vi "Refresh All Hightlight.vi"(0 "Display State In":T1={"logTable"=refnum, "max items"=500, "displaydata"=[], "data"=[], "Auto Scroll"=TRUE, "current item"=500, "col headers"=[], "Add to Top"=TRUE, "Auto resize"=TRUE, "col size"=[], "filters"=[], "color cells"=[]}, 9 "Container State":T3, 11 "error in (no error)":errorcluster) -> (4 "Display State Out":T1={"logTable"=refnum, "max items"=500, "displaydata"=[], "data"=[], "Auto Scroll"=TRUE, "current item"=500, "col headers"=[], "Add to Top"=TRUE, "Auto resize"=TRUE, "col size"=[], "filters"=[], "color cells"=[]}, 15 "error out":errorcluster)   [LabVIEW 2013, in "UI-DisplayTable(dev).xctl"]
uses:
  UI-DisplayTable(dev).xctl
  <vilib>/_xctls/Container State.ctl
  State.ctl
  Support/DEF-Filter.ctl
  <vilib>/Utility/miscctls.llb/LVRowAndColumnTypeDef.ctl
  <vilib>/_xctls/XControlSupport.lvlib
types:
  T1 = typedef "UI-DisplayTable(dev).xctl/State.ctl" = cluster{"logTable":refnum<vi>, "max items":i32, "displaydata":string[][], "data":string[][], "Auto Scroll":bool, "current item":i32, "col headers":string[], "Add to Top":bool, "Auto resize":bool, "col size":i32[], "filters":T2[], "color cells":cluster{"color cell":cluster{"Column":string, "Value":string, "Highlight Column":string}, "Color Box":u32}[]}
  T2 = typedef "UI-DisplayTable(dev).xctl/DEF-Filter.ctl" = cluster{"column":string, "value":string[]}
  T3 = typedef "XControlSupport.lvlib/Container State.ctl" = cluster{"Indicator?":bool, "Run Mode?":bool, " Refnum":refnum<vi>}
  T4 = typedef "LVRowAndColumnTypeDef.ctl" = cluster{"Row":i32, "Column":i32}
  T5 = cluster{"color cell":cluster{"Column":string, "Value":string, "Highlight Column":string}, "Color Box":u32}[]
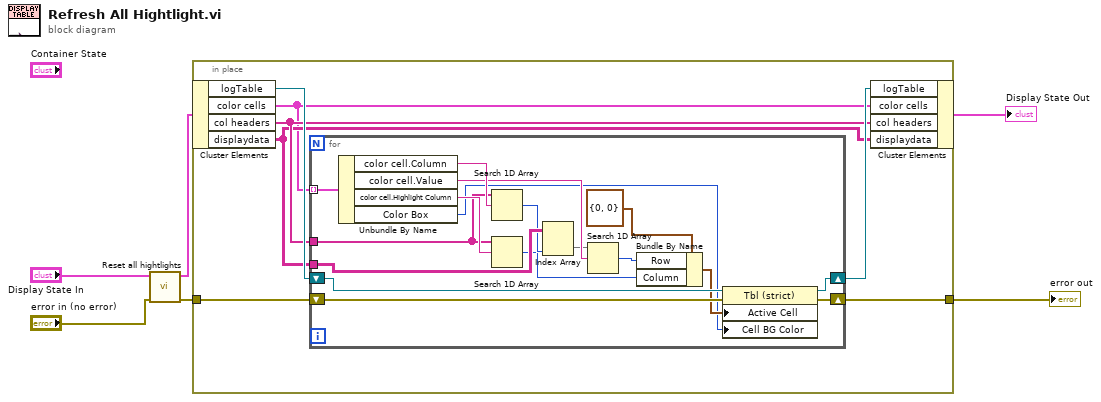
[diagram p0: block diagram]
diagram:
  n1 = call "Reset all hightlights.vi"("error in (no error)"="error in (no error)", "Display State In in"="Display State In") -> ("error out"=w1:errorcluster, "Display State In out"=w3:T1)  [unwired: 8 in]
  n2 = in-place {
    in-place-border: w1 -> [w13]
    in-place-border: [w12] -> w6
    n3 = in-place-cluster #1(w3) -> ("logTable"=w11:refnum<vi>, "color cells"=w7:T5, "col headers"=w9:string[], "displaydata"=w8:string[][])
    n4 = for {
      tunnel: w7 -> [w27] mode=indexing
      shift-right: [w28] -> w12
      shift-left: w13 -> [w29]
      tunnel: w9 -> [w22]
      tunnel: w8 -> [w25]
      shift-right: [w15] -> w10
      shift-left: w11 -> [w30]
      n5 = Unbundle By Name(w27) -> ("color cell.Column"=w26:string, "color cell.Value"=w21:string, "color cell.Highlight Column"=w23:string, "Color Box"=w14:u32)
      n6 = Search 1D Array(1D array=w22, element=w26) -> (index of element=w24:i32)  [unwired: 1 in]
      n7 = Search 1D Array(1D array=w22, element=w23) -> (index of element=w17:i32)  [unwired: 1 in]
      n8 = Index Array(array=w25, index (col)=w24) -> (element=w20:string[])  [unwired: 1 in]
      n9 = Search 1D Array(1D array=w20, element=w21) -> (index of element=w18:i32)  [unwired: 1 in]
      n10 = Bundle By Name(cluster=T4 {"Row"=0, "Column"=0} ("Active Cell:Active Cell"), "Row"=w18, "Column"=w17) -> (w16:T4)
      n11 = property class="Tbl (strict)"(reference=w30, error in=w29, "Active Cell"=w16, "Cell BG Color"=w14) -> (reference out=w15:refnum<vi>, error out=w28:errorcluster)
    }
    n12 = in-place-cluster #1("logTable"=w10, "color cells"=w7, "col headers"=w9, "displaydata"=w8) -> (→"Display State Out":T1)
  }
  "error out" <- w6
